vi "GenerateAllClassLibList.vi"(6 "GUI Mode? {F)":bool, 8 "error in (no error)":errorcluster, 11 "Workspace Path":path=path "E:/sw-deps-monitor") -> (0 "error out":errorcluster)   [LabVIEW 2019, in "Hawkeye.lvlib"]
uses:
  Hawkeye.lvlib
  ead0c1dc-4abe-4fdf-93af-0a2c3e7fff4b.vi
  <vilib>/Wiresmith Technology/G CLI/CLI Class/CLI.lvclass
panel:
  in  "Tab Control":enum32{"GUI Mode", "CLI Mode"}(tab)=enum."CLI Mode"
  out "Args":string[](array[string])=["E:\\sw-deps-monitor"]
  # "When in GUI Mode, the controls will be used, \nin CLI Mode the Args will be used"
  # "Command to run the VI from terminal\n\ng-cli -v --lv-ver 2023 --arch 32 \"E:\\sw-deps-monitor\\CICD\\CheckModifiedVIs\\GenerateAllClassLibList.vi\" -- \"E:\\sw-deps-monitor\""
  # "Workspace Path"
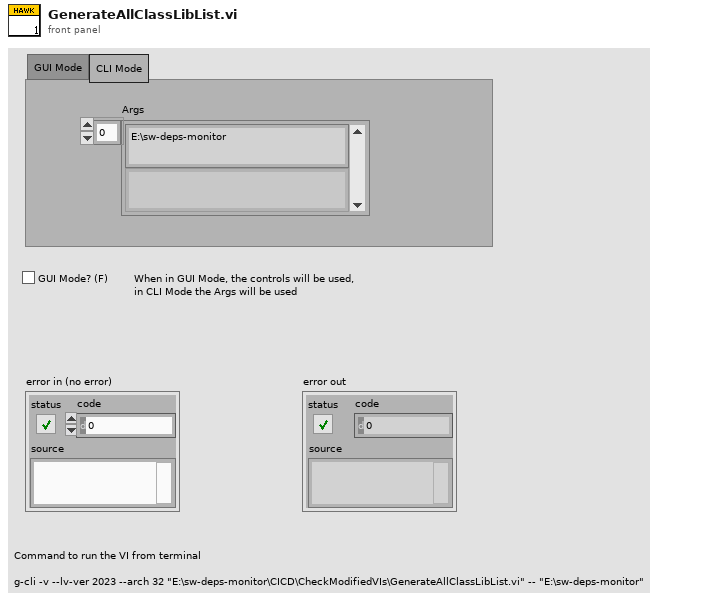
[diagram p1: front panel]
types:
  T1 = enum16{"open", "replace", "create", "open or create", "replace or create", "replace or create with confirmation"}
  T2 = typedef "Hawkeye.lvlib/HawkeyePathConfigs.ctl" = cluster{"GlobalIncludePaths":path[], "GlobalExcludePaths":path[], "BuildSpecsIncludePaths":path[], "ActualDepsIncludePaths":path[], "WorkspacePath":path, "SourceFolderPaths":path[], "ChangedFilesLogpaths":map{string, path}}
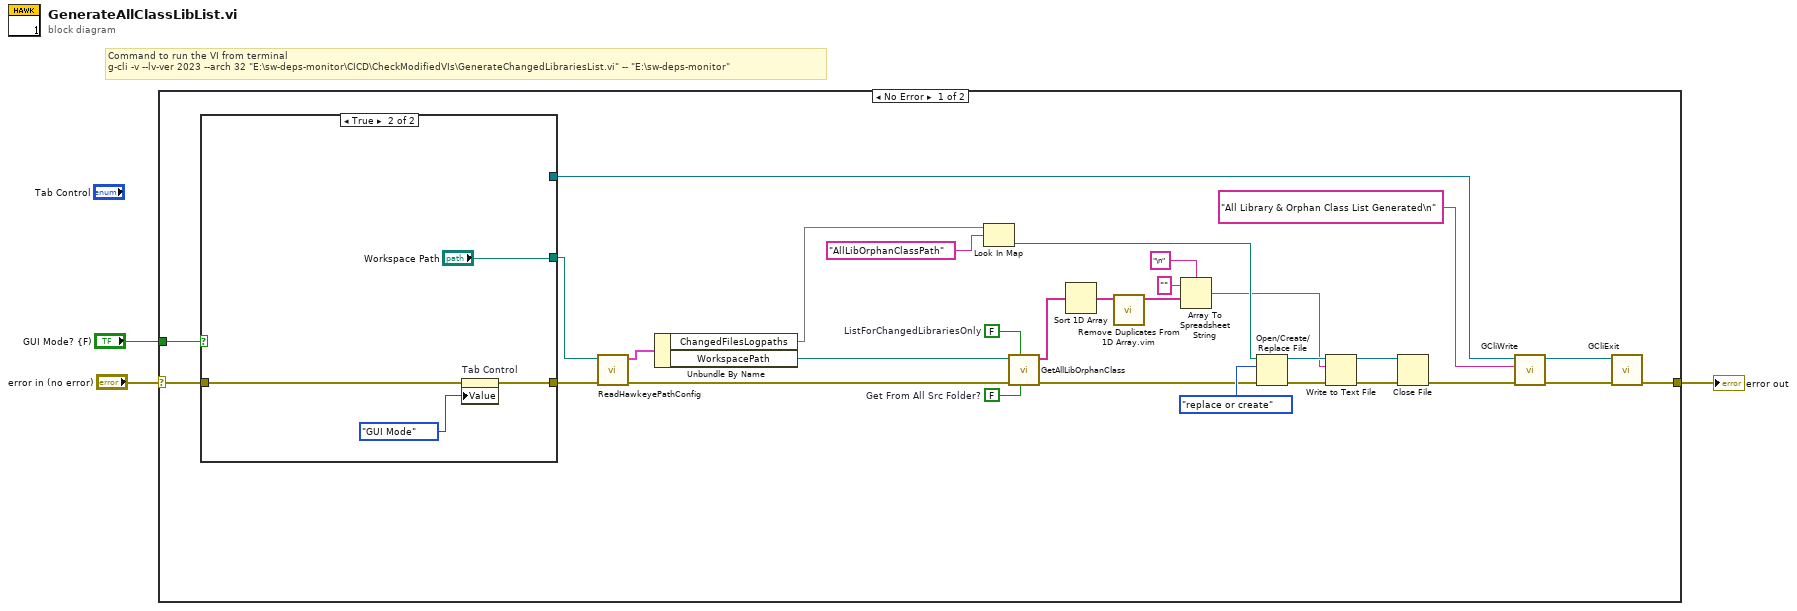
[diagram p0: block diagram]
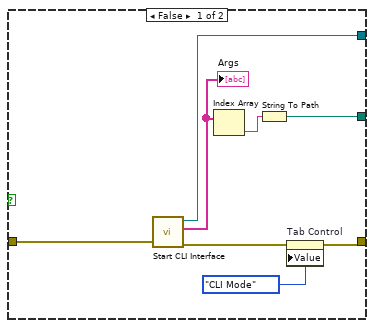
[diagram p2: hidden frame]
diagram:
  # "Command to run the VI from terminal\ng-cli -v --lv-ver 2023 --arch 32 \"E:\\sw-deps-monitor\\CICD\\CheckModifiedVIs\\GenerateChangedLibrariesList.vi\" -- \"E:\\sw-deps-monitor\""
  n1 = case shown="No Error" "error in (no error)" {
    selector: "error in (no error)" -> [w32 w46]
    tunnel: "GUI Mode? {F)" -> [w33 _]
    tunnel: [w29 w46] -> w1
    frame No Error {
      w10 = FALSE  # Get From All Src Folder?
      w11 = FALSE  # ListForChangedLibrariesOnly
      n2 = case shown="True" w33 {
        tunnel: [w40 "Workspace Path"] -> w27
        tunnel: w32 -> [w39 w44]
        tunnel: [w37 w42] -> w26
        tunnel: [w38 _] -> w31
        frame False {
          n3 = call <vilib>:"Start CLI Interface.vi"("error in (no error)"=w39) -> ("error out"=w35:errorcluster, "Custom Parameters"=w34:string[], "CLI out"=w38:refnum<class "CLI.lvclass">)  [unwired: 7 in, 1 out]
          "Args" <- w34
          n4 = Index Array(array=w34) -> (element=w41:string)  [unwired: 1 in]
          n5 = String To Path(string=w41) -> (path=w40:path)
          n6 = property on="Tab Control" class="TabCtl (strict)"(error in=w35, "Value"=enum32{"GUI Mode", "CLI Mode"}."CLI Mode" ("Tab Control")) -> (error out=w37:errorcluster)  [unwired: 1 in, 1 out]
        }
        frame True {
          n7 = property on="Tab Control" class="TabCtl (strict)"(error in=w44, "Value"=enum32{"GUI Mode", "CLI Mode"}."GUI Mode" ("Tab Control")) -> (error out=w42:errorcluster)  [unwired: 1 in, 1 out]
        }
      }
      n8 = call "ReadHawkeyePathConfig.vi"("error in (no error)"=w26, "Workspace Path"=w27) -> ("error out"=w9:errorcluster, "Hawkeye Path Config Out"=w25:T2)  [unwired: 8 in]
      n9 = Unbundle By Name(w25) -> ("ChangedFilesLogpaths"=w23:map{string, path}, "WorkspacePath"=w6:path)
      n10 = Look In Map(map=w23, key="AllLibOrphanClassPath") -> (value=w22:path)  [unwired: 1 in, 1 out]
      n11 = call "GetAllLibOrphanClass.vi"("Get From All Src Folder?"=w10, "ListForChangedLibrariesOnly"=w11, "error in (no error)"=w9, "Workspace Path"=w6) -> ("error out"=w8:errorcluster, "Lib / Class Name []"=w7:string[])  [unwired: 5 in, 1 out]
      n12 = Sort 1D Array(array=w7) -> (sorted array=w4:string[])
      n13 = call "Remove Duplicates From 1D Array.vim"("array"=w4) -> ("array with duplicates removed"=w12:string[])  [unwired: 10 in]
      n14 = Array To Spreadsheet String(delimiter (Tab)="\n", array=w12, 3:"" ("format string")) -> (spreadsheet string=w14:string)
      n15 = Open/Create/Replace File(file path (use dialog)=w22, error in=w8, operation (0:open)=T1."replace or create") -> (refnum out=w19:refnum<file>, error out=w20:errorcluster)  [unwired: 3 in, 1 out]
      n16 = Write to Text File(file (use dialog)=w19, text=w14, error in=w20) -> (refnum out=w17:refnum<file>, error out=w18:errorcluster)  [unwired: 1 in, 1 out]
      n17 = Close File(refnum=w17, error in=w18) -> (error out=w13:errorcluster)  [unwired: 1 out]
      n18 = call "GCliWrite.vi"("error in (no error)"=w13, "Text to Write"="All Library & Orphan Class List Generated\n", "CLI in"=w31) -> ("error out"=w30:errorcluster, "CLI out"=w28:refnum<class "CLI.lvclass">)  [unwired: 7 in]
      n19 = call "GCliExit.vi"("error in (no error)"=w30, "CLI in"=w28) -> ("error out"=w29:errorcluster)  [unwired: 9 in]
    }
    frame Error {
    }
  }
  "error out" <- w1
